vi "Create_DAQ_Time_Axis.vi"(6 "NOT [Last Data Point Dumped?]":bool=TRUE, 7 "Time Stamp Current Iteration":timestamp, 9 "Time Stamp Last Iteration":timestamp, 11 "Time Array IN":dbl[](array[numeric])) -> (1 "Time Stamp Current Iteration":timestamp, 2 "Loop Time (ms)":u32, 3 "Time Array OUT":dbl[](array[numeric]))   [LabVIEW 2018]
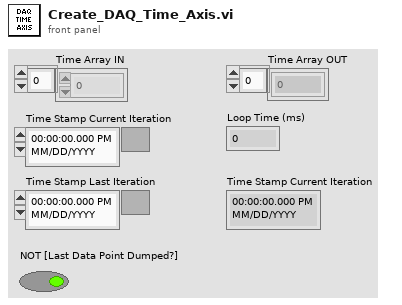
[diagram p1: front panel]
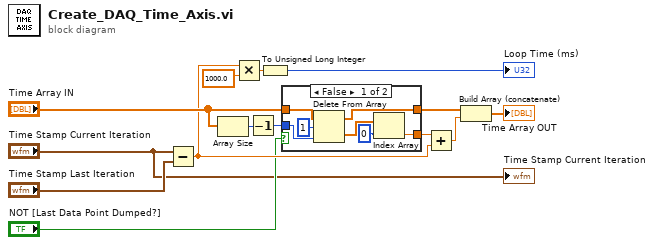
[diagram p0: block diagram]
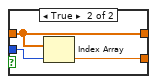
[diagram p2: hidden frame]
diagram:
  n1 = Subtract(x="Time Stamp Current Iteration", y="Time Stamp Last Iteration") -> (x-y=w4:dbl)
  n2 = Array Size(array="Time Array IN") -> (size(s)=w14:i32)
  n3 = Multiply(x=w4, y=1000.0) -> (x*y=w11:dbl)
  n4 = Decrement(x=w14) -> (x-1=w9:i32)
  n5 = To Unsigned Long Integer(number=w11) -> (unsigned 32bit integer=→"Loop Time (ms)":u32)
  n6 = case shown="False" "NOT [Last Data Point Dumped?]" {
    tunnel: "Time Array IN" -> [w21 w24]
    tunnel: [w18 w24] -> w7
    tunnel: w9 -> [w19 w23]
    tunnel: [w15 w22] -> w8
    frame False {
      n7 = Delete From Array(array=w21, length=1, index=w19) -> (deleted portion=w17:dbl[], array with subset deleted=w18:dbl[])
      n8 = Index Array(array=w17, index=0) -> (element=w15:dbl)
    }
    frame True {
      n9 = Index Array(array=w24, index=w23) -> (element=w22:dbl)
    }
  }
  n10 = Add(x=w8, y=w4) -> (x+y=w13:dbl)
  n11 = Build Array (concatenate)(w7, w13) -> (→"Time Array OUT":dbl[])
  "Time Stamp Current Iteration" <- "Time Stamp Current Iteration"
